vi "onWriteMapping.vi"(8 "error in (no error)":errorcluster, 9 "TestCaseMap":map{string, set{string}}(c390), 10 "RequirementMap":map{string, set{string}}(c390), 11 "Pips.TestResults in":refnum<class "Pips.TestResults.lvclass">) -> (0 "error out":errorcluster, 3 "Pips.TestResults out":refnum<class "Pips.TestResults.lvclass">)   [LabVIEW 2021, in "Banana.Caraya.lvlib" / "Pips.TestResults.lvclass"]
uses:
  Pips.TestResults.lvclass
  Pips.TestResults.lvclass/Pips.TestResults.ctl
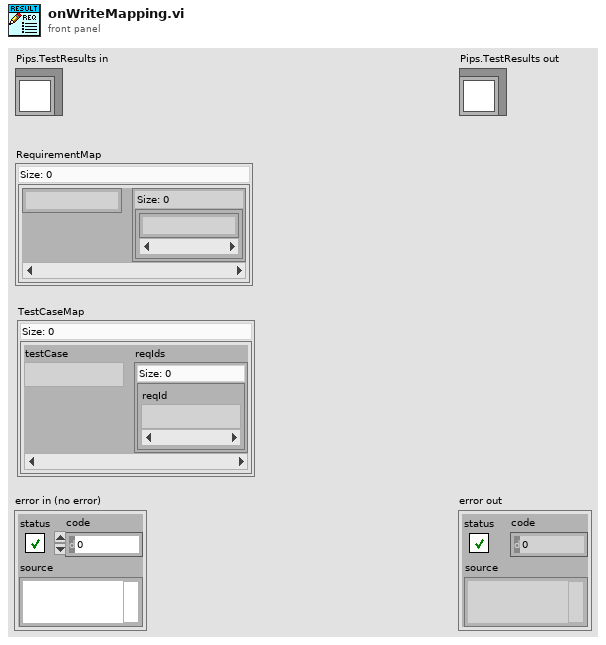
[diagram p1: front panel]
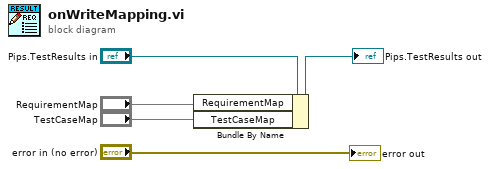
[diagram p0: block diagram]
diagram:
  n1 = Bundle By Name(cluster="Pips.TestResults in", "RequirementMap"="RequirementMap", "TestCaseMap"="TestCaseMap") -> (→"Pips.TestResults out":refnum<class "Pips.TestResults.lvclass">)
  "error out" <- "error in (no error)"
